vi "TharInit.vi"(8 "error in (no error)":errorcluster, 11 "configuration file path":path) -> (0 "Error Out":errorcluster, 2 "serial":string)   [LabVIEW 2016]
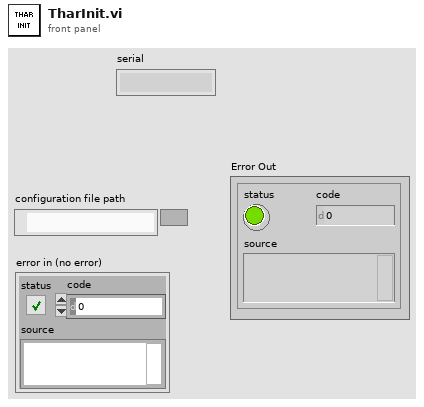
[diagram p1: front panel]
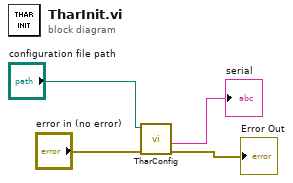
[diagram p0: block diagram]
diagram:
  n1 = call "TharConfig.vi"("Error In"="error in (no error)", "configuration file path"="configuration file path") -> ("Error Out"=→"Error Out":errorcluster, "serial"=→"serial":string)  [unwired: 6 in, 2 out]
